vi "Laser Tester.vi"() -> ()   [LabVIEW 2017]
panel:
  in  "Laser On/Off":bool
  in  "Laser Power (mW)":dbl min=0.0 max=120.0 step=1.0
  in  "stop":bool
  in  "Laser to initialise":string(combo)
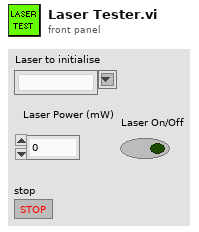
[diagram p1: front panel]
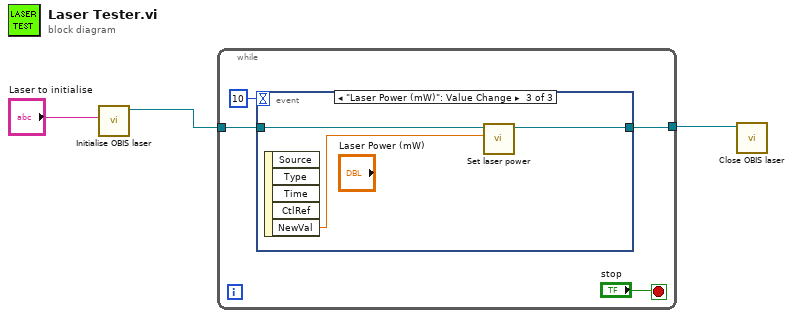
[diagram p0: block diagram]
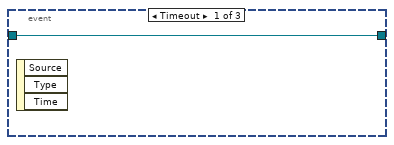
[diagram p2: hidden frame]
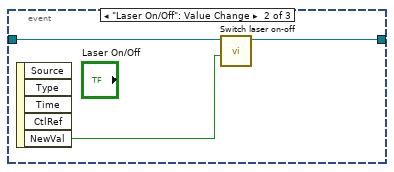
[diagram p3: hidden frame]
diagram:
  n1 = call "Initialise OBIS laser.vi"("Laser to initialise"="Laser to initialise") -> ("VISA resource name out"=w2:refnum<visa-resource-name>)  [unwired: 8 in, 2 out]
  n2 = while {
    tunnel: w2 -> [w6]
    tunnel: [w5] -> w1
    stop <- "stop" stop-if-true
    n3 = event shown="[2] \"Laser Power (mW)\": Value Change" {
      selector: _ -> [_ _ _]
      dyn-events: _ -> [_ _ _]
      timeout: 10 -> [_ _ _]
      tunnel: w6 -> [w8 w11 w14]
      tunnel: [w8 w10 w13] -> w5
      event Timeout {
        n4 = event-data() -> ()  [unwired: 1 in, 3 out]
      }
      event "Laser On/Off": Value Change {
        n5 = event-data() -> ("NewVal"=w9:bool)  [unwired: 1 in, 4 out]
        n6 = call "Switch laser on-off.vi"("Laser On/Off"=w9, "VISA resource name"=w11) -> ("VISA resource name out"=w10:refnum<visa-resource-name>)  [unwired: 9 in]
      }
      event "Laser Power (mW)": Value Change {
        n7 = event-data() -> ("NewVal"=w12:dbl)  [unwired: 1 in, 4 out]
        n8 = call "Set laser power.vi"("Laser Power"=w12, "VISA resource name"=w14) -> ("VISA resource name out"=w13:refnum<visa-resource-name>)  [unwired: 9 in]
      }
    }
  }
  n9 = call "Close OBIS laser.vi"("VISA resource name"=w1) -> ()  [unwired: 10 in, 1 out]
